vi "Part 2.vi"(11 "Input":string) -> (3 "Output":i64)   [LabVIEW 2021]
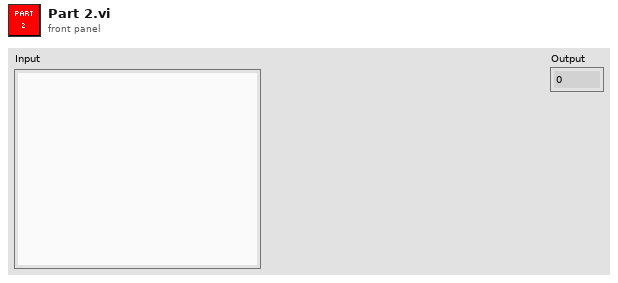
[diagram p1: front panel]
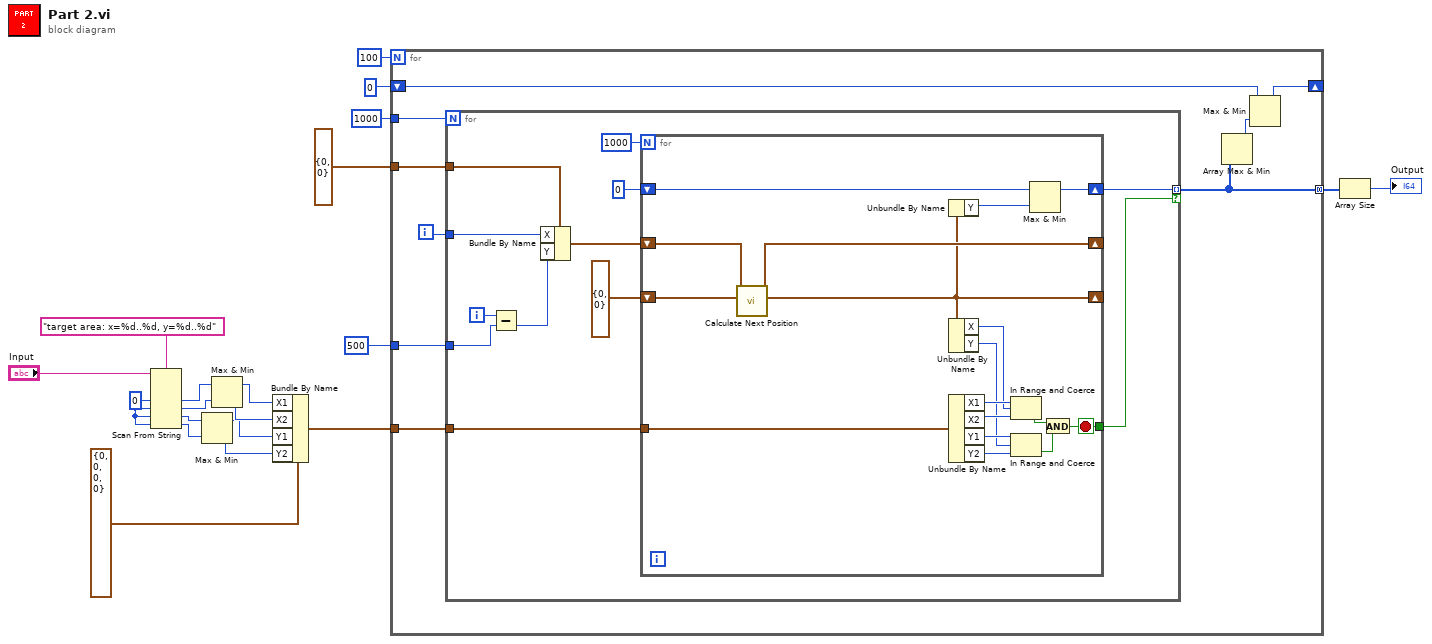
[diagram p0: block diagram]
diagram:
  w5 = i64 0 ("default value 1")
  n1 = Scan From String(format string="target area: x=%d..%d, y=%d..%d", input string="Input", default 1=w5, default 2=w5, default 3=w5, default 4=w5) -> (output 1=w15:i64, output 2=w13:i64, output 3=w11:i64, output 4=w9:i64)  [unwired: 2 in, 3 out]
  n2 = Max & Min(x=w11, y=w9) -> (max(x,y)=w10:i64, min(x,y)=w8:i64)
  n3 = Max & Min(x=w15, y=w13) -> (max(x,y)=w14:i64, min(x,y)=w12:i64)
  n4 = Bundle By Name(cluster=cluster{"X1":i64, "X2":i64, "Y1":i64, "Y2":i64} {"X1"=0, "X2"=0, "Y1"=0, "Y2"=0}, "X1"=w14, "X2"=w12, "Y1"=w10, "Y2"=w8) -> (w16:cluster{"X1":i64, "X2":i64, "Y1":i64, "Y2":i64})
  n5 = for {
    N: 100 -> [_]
    tunnel: 1000 -> [w29]
    tunnel: w16 -> [w28]
    tunnel: cluster{"X":i64, "Y":i64} {"X"=0, "Y"=0} -> [w27]
    tunnel: [w25] -> w7 mode=concatenating
    shift-right: [w22] -> _
    shift-left: i64 0 -> [w23]
    tunnel: 500 ("y") -> [w21]
    i -> [w26]
    n6 = for {
      N: w29 -> [_]
      tunnel: w28 -> [w41]
      tunnel: w27 -> [w40]
      tunnel: w26 -> [w39]
      tunnel: [w35] -> w25 mode=indexing if=w34
      tunnel: w21 -> [w30]
      i -> [w31]
      n7 = Subtract(x=w31, y=w30) -> (x-y=w32:i32)
      n8 = Bundle By Name(cluster=w40, "X"=w39, "Y"=w32) -> (w38:cluster{"X":i64, "Y":i64})
      n9 = for {
        N: 1000 -> [_]
        tunnel: w41 -> [w58]
        shift-right: [w42] -> _
        shift-left: cluster{"X":i64, "Y":i64} {"X"=0, "Y"=0} -> [w45]
        shift-right: [w43] -> _
        shift-left: w38 -> [w44]
        shift-right: [w47] -> w35
        shift-left: i64 0 -> [w48]
        tunnel: [w46] -> w34
        stop <- w46 stop-if-true
        n10 = call "Calculate Next Position.vi"("Position In"=w45, "Velocity In"=w44) -> ("Position Out"=w42:cluster{"X":i64, "Y":i64}, "Velocity Out"=w43:cluster{"X":i64, "Y":i64})  [unwired: 8 in]
        n11 = Unbundle By Name(w42) -> ("Y"=w49:i64)
        n12 = Unbundle By Name(w42) -> ("X"=w55:i64, "Y"=w52:i64)
        n13 = Unbundle By Name(w58) -> ("X1"=w57:i64, "X2"=w56:i64, "Y1"=w54:i64, "Y2"=w53:i64)
        n14 = In Range and Coerce(upper limit=w57, x=w55, lower limit=w56) -> (In Range?=w51:bool)  [unwired: 1 out]
        n15 = In Range and Coerce(upper limit=w54, x=w52, lower limit=w53) -> (In Range?=w50:bool)  [unwired: 1 out]
        n16 = Max & Min(x=w48, y=w49) -> (max(x,y)=w47:i64)  [unwired: 1 out]
        n17 = And(x=w51, y=w50) -> (x .and. y?=w46:bool)
      }
    }
    n18 = Array Max & Min(array=w25) -> (max value=w24:i64)  [unwired: 3 out]
    n19 = Max & Min(x=w23, y=w24) -> (max(x,y)=w22:i64)  [unwired: 1 out]
  }
  n20 = Array Size(array=w7) -> (size(s)=→"Output":i32)
